vi "StopEqualization.vi"(8 "error in (no error)":errorcluster, 11 "reference in":refnum<class "mmWave instrument.lvclass">) -> (0 "error out":errorcluster, 3 "reference out":refnum<class "mmWave instrument.lvclass">)   [LabVIEW 2019, in "mmWave instrument.lvclass"]
doc: "Stops equalization procedure"
uses:
  mmWave instrument.lvclass
  Instrument state.ctl
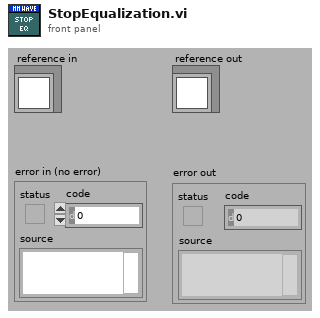
[diagram p1: front panel]
types:
  T1 = typedef "mmWave instrument.lvclass/Instrument state.ctl" = enum16{"Off", "Initialization", "Configuration", "Running", "Calibration"}
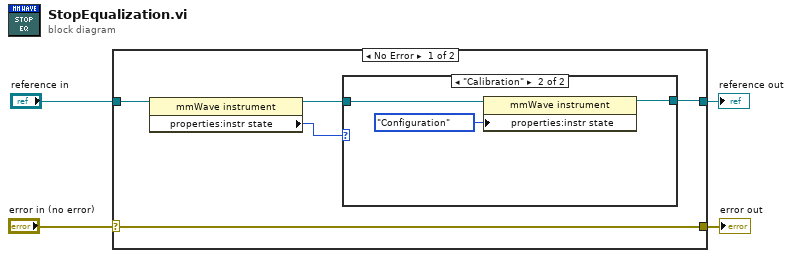
[diagram p0: block diagram]
diagram:
  n1 = case shown="No Error" "error in (no error)" {
    selector: "error in (no error)" -> [w9 w15]
    tunnel: [w9 w15] -> w3
    tunnel: [w5 w14] -> w1
    tunnel: "reference in" -> [w8 w14]
    frame No Error {
      n2 = property class="mmWave instrument"(reference=w8) -> (reference out=w6:refnum<class "mmWave instrument.lvclass">, "properties:instr state"=w7:T1)  [unwired: 1 in, 1 out]
      n3 = case shown="\"Calibration\"" w7 {
        tunnel: w6 -> [w10 w13]
        tunnel: [w10 w12] -> w5
        frame "Off", Default {
        }
        frame "Calibration" {
          n4 = property class="mmWave instrument"(reference=w13, "properties:instr state"=Instrument_state."Configuration" ("instr state")) -> (reference out=w12:refnum<class "mmWave instrument.lvclass">)  [unwired: 1 in, 1 out]
        }
      }
    }
    frame Error {
    }
  }
  "error out" <- w3
  "reference out" <- w1
